vi "Periodic Tasks.vi"(8 "error in":errorcluster) -> ()   [LabVIEW 2018]
doc: "This VI runs in parallel to other tasks. It can contain as many user-defined periodic loops as you need. These can carry out PID or other sorts of timed response."
uses:
  LeftMotors.ctl
  RightMotors.ctl
  <vilib>/Rock Robotics/WPI/ThirdParty/Phoenix-LabVIEW/Motor Controller/Controls/CTRE_Phoenix_MotorControl_ControlMode.ctl
panel:
  in  "stop":bool
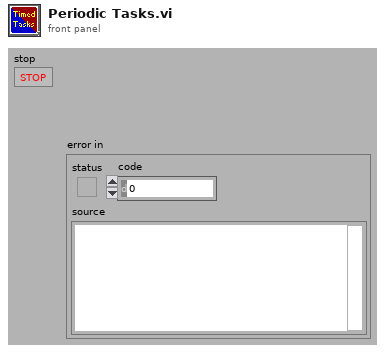
[diagram p1: front panel]
types:
  T1 = typedef "RightMotors.ctl" = enum16{"Right Motor 1", "Right Motor 2", "Right Motor 3"}
  T2 = typedef "LeftMotors.ctl" = enum16{"LeftMotor1", "LeftMotor2", "LeftMotor3"}
  T3 = typedef "WPI_MotorControlDeviceRef.ctl" = cluster{"DeviceStatus":errorcluster, "Type":T4, "PWM":cluster{"PWM Channel":T5, "DeadBand":T6}, "CAN":cluster{"Device Number":u8, "SetOutput VI Ref":variant, "GetOutput VI Ref":variant, "Enable VI Ref":variant, "Disable VI Ref":variant, "Data":variant}, "Invert":bool, "DIO PWM":cluster{"PWM \"Enable\" Channel":T5, "DIOChannel":T7, "PWM Rate":dbl}}
  T4 = typedef "WPI_MotorControlType.ctl" = enum16{"PWM", "CAN", "DIO PWM"}
  T5 = typedef "FPGA_DIOPWMChannel.ctl" = enum8{"PWM 0", "PWM 1", "PWM 2", "PWM 3", "PWM 4", "PWM 5", "PWM 6", "PWM 7", "PWM 8", "PWM 9", "PWM MXP 0", "PWM MXP 1", "PWM MXP 2", "PWM MXP 3", "PWM MXP 4", "PWM MXP 5", "PWM MXP 6", "PWM MXP 7", "PWM MXP 8", "PWM MXP 9", "Invalid"}
  T6 = typedef "WPI_PWMDeadband.ctl" = cluster{"Name":string, "maxPositivePwm":i32, "minPositivePwm":i32, "centerPwm":i32, "maxNegativePwm":i32, "minNegativePwm":i32, "angularRange":u16}
  T7 = typedef "FPGA_DIOChannel.ctl" = enum8{"DIO 0", "DIO 1", "DIO 2", "DIO 3", "DIO 4", "DIO 5", "DIO 6", "DIO 7", "DIO 8", "DIO 9", "DIO MXP 0", "DIO MXP 1", "DIO MXP 2", "DIO MXP 3", "DIO MXP 4", "DIO MXP 5", "DIO MXP 6", "DIO MXP 7", "DIO MXP 8", "DIO MXP 9", "DIO MXP 10", "DIO MXP 11", "DIO MXP 12", "DIO MXP 13", "DIO MXP 14", "DIO MXP 15", "SPI Port CS1", "SPI Port CS2", "SPI Port CS3", "SPI Port MISO", "SPI Port MOSI", "Invalid"}
  T8 = typedef "CTRE_Phoenix_MotorControl_ControlMode.ctl" = u16
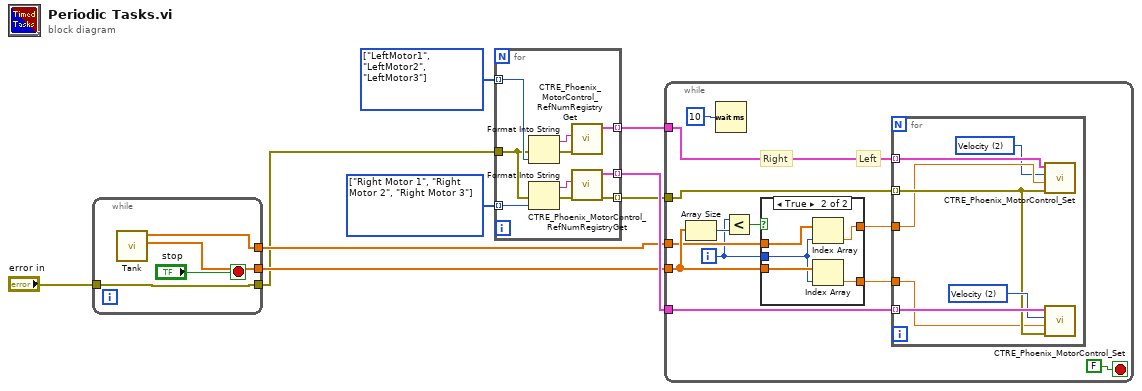
[diagram p0: block diagram]
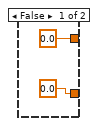
[diagram p2: hidden frame]
diagram:
  w8 = T1[] [enum."Right Motor 1", enum."Right Motor 2", enum."Right Motor 3"] items=["Right Motor 1", "Right Motor 2", "Right Motor 3"] ("Array")
  w9 = T2[] [enum."LeftMotor1", enum."LeftMotor2", enum."LeftMotor3"] items=["LeftMotor1", "LeftMotor2", "LeftMotor3"] ("Array")
  n1 = while {
    tunnel: [w13] -> w4
    tunnel: [w11] -> w3
    tunnel: "error in" -> [w12]
    tunnel: [w12] -> w1
    stop <- "stop" stop-if-true
    n2 = call "Tank.vi"() -> ("right velocity"=w13:dbl[], "left velocity"=w11:dbl[])  [unwired: 10 in]
  }
  n3 = for {
    tunnel: w9 -> [w23] mode=indexing
    tunnel: w8 -> [w21] mode=indexing
    tunnel: w1 -> [w18]
    tunnel: [w16] -> w7 mode=indexing
    tunnel: [w15] -> w6 mode=indexing
    tunnel: [w14] -> w5 mode=indexing
    n4 = Format Into String(error in=w18, w23) -> (resulting string=w22:string, error out=w19:errorcluster)  [unwired: 2 in]
    n5 = Format Into String(error in=w18, w21) -> (resulting string=w20:string, error out=w17:errorcluster)  [unwired: 2 in]
    n6 = call <vilib>:"CTRE_Phoenix_MotorControl_RefNumRegistryGet.vi"("error in (no error)"=w19, "refnum name"=w22) -> ("PhoenixMotorControlDevRef"=w16:T3)  [unwired: 8 in, 1 out]
    n7 = call <vilib>:"CTRE_Phoenix_MotorControl_RefNumRegistryGet.vi"("error in (no error)"=w17, "refnum name"=w20) -> ("error out"=w14:errorcluster, "PhoenixMotorControlDevRef"=w15:T3)  [unwired: 8 in]
  }
  n8 = while {
    tunnel: w7 -> [w34]
    tunnel: w6 -> [w33]
    tunnel: w5 -> [w32]
    tunnel: w4 -> [w28]
    tunnel: w3 -> [w27]
    i -> [w26]
    stop <- FALSE stop-if-true
    # "Right"
    # "Left"
    n9 = Array Size(array=w28) -> (size(s)=w29:i32)
    n10 = Wait (ms)(milliseconds to wait=u32 10) -> ()  [unwired: 1 out]
    n11 = Less?(x=w26, y=w29) -> (x < y?=w30:bool)
    n12 = case shown="True" w30 {
      tunnel: w28 -> [_ w42]
      tunnel: w27 -> [_ w41]
      tunnel: w26 -> [_ w40]
      tunnel: [0.0 ("velocity") w39] -> w25
      tunnel: [0.0 ("velocity") w38] -> w24
      frame False {
      }
      frame True {
        n13 = Index Array(array=w41, index=w40) -> (element=w39:dbl)
        n14 = Index Array(array=w42, index=w40) -> (element=w38:dbl)
      }
    }
    n15 = for {
      tunnel: w34 -> [w49] mode=indexing
      tunnel: w33 -> [w48] mode=indexing
      tunnel: w32 -> [w46] mode=indexing
      tunnel: w25 -> [w45]
      tunnel: w24 -> [w44]
      w47 = T8 2 items=["PercentOutput"=0, "Position"=1, "Velocity"=2, "Current"=3, "Follower"=5, "MotionProfile"=6, "MotionMagic"=7, "MotionProfileArc"=10, "Disabled"=15] ("Control Mode")
      w43 = T8 2 items=["PercentOutput"=0, "Position"=1, "Velocity"=2, "Current"=3, "Follower"=5, "MotionProfile"=6, "MotionMagic"=7, "MotionProfileArc"=10, "Disabled"=15] ("Control Mode")
      n16 = call <vilib>:"CTRE_Phoenix_MotorControl_Set.vi"("error in (no error)"=w46, "Output"=w45, "Control Mode"=w43, "PhoenixMotorControlDevRef"=w49) -> ()  [unwired: 6 in, 2 out]
      n17 = call <vilib>:"CTRE_Phoenix_MotorControl_Set.vi"("error in (no error)"=w46, "Output"=w44, "Control Mode"=w47, "PhoenixMotorControlDevRef"=w48) -> ()  [unwired: 6 in, 2 out]
    }
  }
